vi "toStringArray.vi"(8 "error in (no error)":errorcluster, 11 "RampTone in":refnum<class "RampTone.lvclass">) -> (0 "error out":errorcluster, 2 "eventStringArray":string[](array[string]), 3 "RampTone out":refnum<class "RampTone.lvclass">)   [LabVIEW 2009, in "Tools.lvlib" / "Scripting.lvlib" / "RampTone.lvclass"]
uses:
  RampTone.lvclass
  SingleTone/SingleTone.lvclass
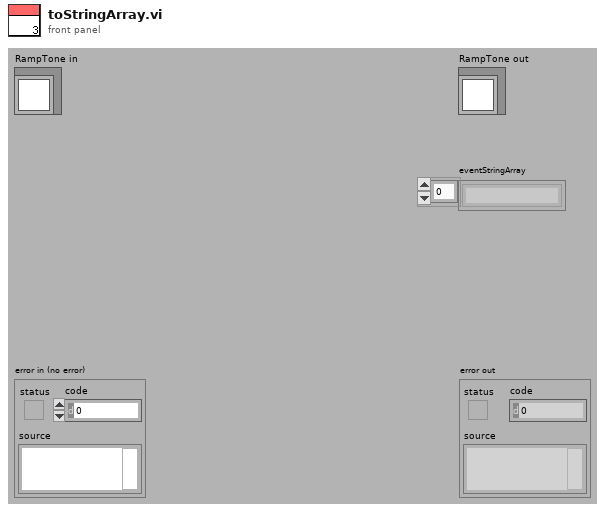
[diagram p1: front panel]
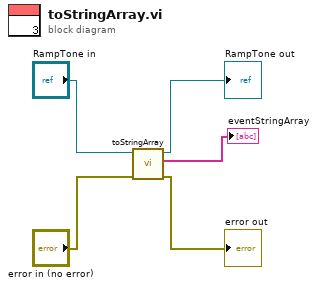
[diagram p0: block diagram]
diagram:
  n1 = call-parent "toStringArray.vi"("error in (no error)"="error in (no error)", "SingleTone in"="RampTone in") -> ("error out"=→"error out":errorcluster, "eventStringArray"=→"eventStringArray":string[], "SingleTone out"=→"RampTone out":refnum<class "RampTone.lvclass">)  [unwired: 7 in]
